vi "Open_COM.vi"(8 "error in (no error)":errorcluster, 11 "USB-87Pn_Data In":T1) -> (0 "error out":errorcluster, 3 "USB-87Pn_Data Out":T1)   [LabVIEW 2019, in "USB-87P8_Manager.lvlib"]
uses:
  Module/USB-87P8_Manager.lvlib
  USB-87Pn_Data.ctl
  USB-87Pn.lvclass
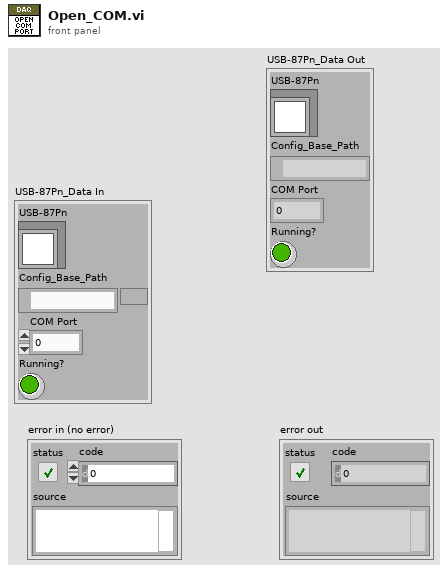
[diagram p1: front panel]
types:
  T1 = typedef "USB-87P8_Manager.lvlib/USB-87Pn_Data.ctl" = cluster{"USB-87Pn":refnum<class "USB-87Pn.lvclass">, "Config_Base_Path":path, "COM Port":i32, "Running?":bool}
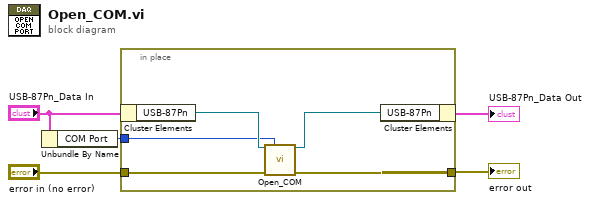
[diagram p0: block diagram]
diagram:
  n1 = Unbundle By Name("USB-87Pn_Data In") -> ("COM Port"=w1:i32)
  n2 = in-place {
    in-place-border: "error in (no error)" -> [w10]
    in-place-border: [w7] -> w3
    in-place-border: w1 -> [w6]
    n3 = in-place-cluster #1("USB-87Pn_Data In") -> ("USB-87Pn"=w9:refnum<class "USB-87Pn.lvclass">)
    n4 = call "Open_COM.vi"("USB-87Pn in"=w9, "port number"=w6, "error in (no error)"=w10) -> ("USB-87Pn out"=w8:refnum<class "USB-87Pn.lvclass">, "error out"=w7:errorcluster)  [unwired: 11 in]
    n5 = in-place-cluster #1("USB-87Pn"=w8) -> (→"USB-87Pn_Data Out":T1)
  }
  "error out" <- w3
